vi "Set Property.vi"(8 "error in (no error)":errorcluster, 9 "Value":dbl, 10 "Property":string, 11 "File in":refnum<class "File.lvclass">) -> (0 "error out":errorcluster, 3 "File out":refnum<class "File.lvclass">)   [LabVIEW 2020, in "File.lvclass"]
uses:
  File.lvclass
  File.lvclass/File.ctl
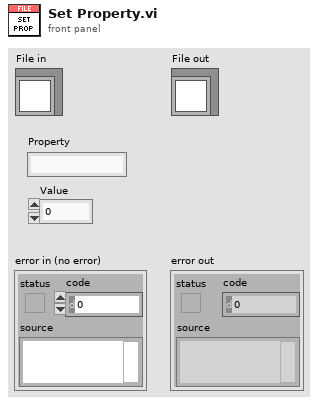
[diagram p1: front panel]
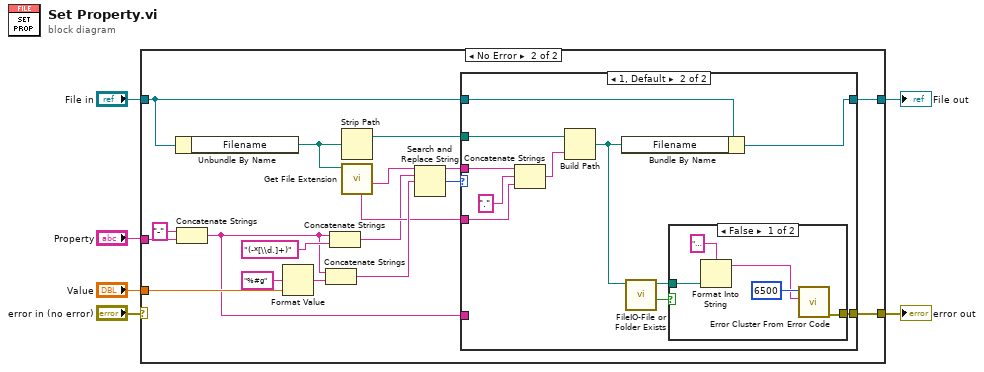
[diagram p0: block diagram]
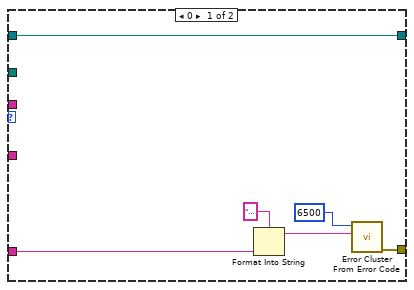
[diagram p3: hidden frame]
diagram:
  n1 = case shown="No Error" "error in (no error)" {
    selector: "error in (no error)" -> [w7 _]
    tunnel: "File in" -> [w8 w13]
    tunnel: [w8 w12] -> w4
    tunnel: "Property" -> [_ w26]
    tunnel: "Value" -> [_ w15]
    tunnel: [w7 w14] -> w1
    frame Error {
    }
    frame No Error {
      n2 = Unbundle By Name(w13) -> ("Filename"=w19:path)
      n3 = Concatenate Strings("-" ("string"), w26) -> (w9:string)
      n4 = Format Value(format string="%#g", value (0)=w15) -> (output string=w23:string)  [unwired: 1 in]
      n5 = Concatenate Strings(w9, w23) -> (w21:string)
      n6 = Concatenate Strings(w9, "(-*[\\d.]+)" ("string")) -> (w10:string)
      n7 = Strip Path(path=w19) -> (stripped path=w18:path)  [unwired: 1 out]
      n8 = call <vilib>:"Get File Extension.vi"("file"=w19) -> ("filename without extension"=w20:string, "unmodified file extension"=w16:string)  [unwired: 6 in, 3 out]
      n9 = Search and Replace String(input string=w20, search string=w10, replace string=w21) -> (result string=w17:string, number of replacements=w11:i32)  [unwired: 5 in, 2 out]
      n10 = case shown="1, Default" w11 {
        tunnel: w18 -> [_ w43]
        tunnel: w17 -> [_ w42]
        tunnel: w16 -> [_ w40]
        tunnel: [w28 w38] -> w14
        tunnel: w13 -> [w32 w34]
        tunnel: [w32 w33] -> w12
        tunnel: w9 -> [w27 _]
        frame 0 {
          n11 = Format Into String(format string="Tag not found in filename: %s" ("error message (\"\")"), w27) -> (resulting string=w29:string)  [unwired: 2 in, 1 out]
          n12 = call <vilib>:"Error Cluster From Error Code.vi"("error message (\"\")"=w29, "error code (0)"=6500) -> ("error out"=w28:errorcluster)  [unwired: 7 in]
        }
        frame 1, Default {
          n13 = Concatenate Strings(w42, "." ("string"), w40) -> (w41:string)
          n14 = Build Path(base path=w43, name or relative path=w41) -> (appended path=w36:path)
          n15 = Bundle By Name(cluster=w34, "Filename"=w36) -> (w33:refnum<class "File.lvclass">)
          n16 = call "FileIO-File or Folder Exists.vi"("path"=w36) -> ("Exists?"=w37:bool, "dup path"=w35:path)  [unwired: 7 in, 2 out]
          n17 = case shown="False" w37 {
            tunnel: [w48 _] -> w38
            tunnel: w35 -> [w44 _]
            frame False {
              n18 = Format Into String(format string="File not found: %s" ("error message (\"\")"), w44) -> (resulting string=w45:string)  [unwired: 2 in, 1 out]
              n19 = call <vilib>:"Error Cluster From Error Code.vi"("error message (\"\")"=w45, "error code (0)"=6500) -> ("error out"=w48:errorcluster)  [unwired: 7 in]
            }
            frame True {
            }
          }
        }
      }
    }
  }
  "error out" <- w1
  "File out" <- w4
